vi "4_Checksum_SubVI.vi"(1 "data in":string) -> (0 "x != y?":bool)   [LabVIEW 2024]
panel:
  out "(hi.lo)":u16
  out "sum":u16 format="%04x"
  out "subarray 2":u16[](array[numeric]) format="%02x"
  out "subarray":u16[](array[numeric]) format="%02x"
  out "size(s)":i32
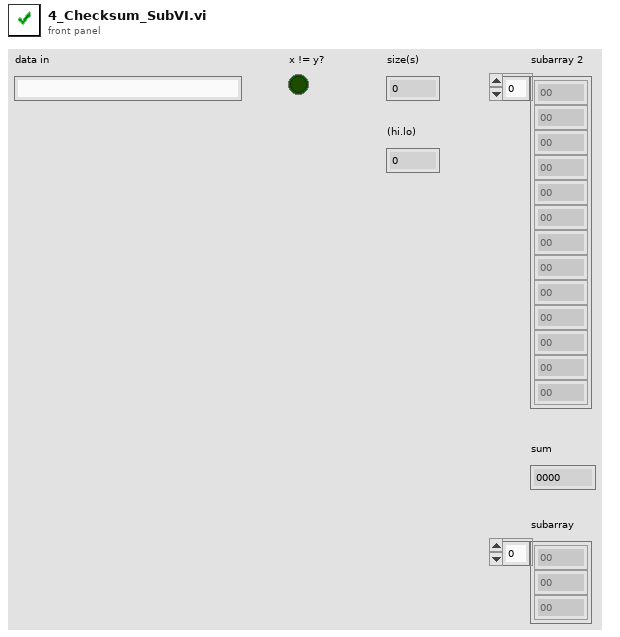
[diagram p1: front panel]
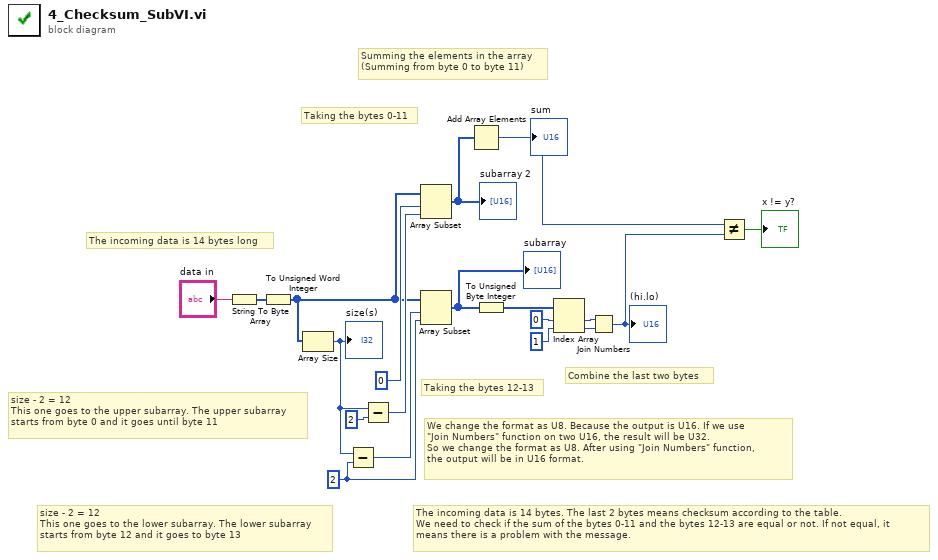
[diagram p0: block diagram]
diagram:
  w3 = 2 ("length")
  # "Combine the last two bytes"
  # "We change the format as U8. Because the output is U16. If we use \n\"Join Numbers\" function on two U16, the result will be U32. \nSo we change the format as U8. After using \"Join Numbers\" function,\nthe output will be in U16 format."
  # "The incoming data is 14 bytes. The last 2 bytes means checksum according to the table.\nWe need to check if the sum of the bytes 0-11 and the bytes 12-13 are equal or not. If not equal, it\nmeans there is a problem with the message."
  # "Taking the bytes 12-13"
  # "size - 2 = 12\nThis one goes to the lower subarray. The lower subarray\nstarts from byte 12 and it goes to byte 13"
  # "size - 2 = 12\nThis one goes to the upper subarray. The upper subarray\nstarts from byte 0 and it goes until byte 11"
  # "The incoming data is 14 bytes long"
  # "Taking the bytes 0-11"
  # "Summing the elements in the array\n(Summing from byte 0 to byte 11)"
  n1 = String To Byte Array(string="data in") -> (unsigned byte array=w2:u8[])
  n2 = To Unsigned Word Integer(number=w2) -> (unsigned 16bit integer=w5:u16[])
  n3 = Array Size(array=w5) -> (size(s)=w6:i32)
  "size(s)" <- w6
  n4 = Subtract(x=w6, y=w3) -> (x-y=w4:i32)
  n5 = Subtract(x=w6, y=2) -> (x-y=w8:i32)
  n6 = Array Subset "Array Subset"(array=w5, index=0, length=w8) -> (w10:u16[])
  "subarray 2" <- w10
  n7 = Array Subset "Array Subset"(array=w5, index=w4, length=w3) -> (w11:u16[])
  "subarray" <- w11
  n8 = Add Array Elements(numeric array=w10) -> (sum=w18:u16)
  "sum" <- w18
  n9 = To Unsigned Byte Integer(number=w11) -> (unsigned 8bit integer=w12:u8[])
  n10 = Index Array "Index Array"(array=w12, index #1=0 ("index"), index #2=1 ("index")) -> (element #1=w15:u8, element #2=w16:u8)
  n11 = Join Numbers(hi=w15, lo=w16) -> ((hi.lo)=w17:u16)
  "(hi.lo)" <- w17
  n12 = Not Equal?(x=w18, y=w17) -> (x != y?=→"x != y?":bool)
